vi "HEWH Agilent Create Label Array.vi"(8 "Error In":errorcluster, 9 "Agilent Calibrated Cluster Array":T1, 10 "Agilent Raw Cluster Array":T1, 11 "Label Array In":string[](array[string])) -> (0 "Error Out":errorcluster, 1 "Agilent Raw Cluster Array Out":T1, 2 "Agilent Calibrated Cluster Array In":T1, 3 "Label Array Out":string[](array[string]))   [LabVIEW 2016]
uses:
  Type Definitions/HEWH Agilent Cluster.ctl
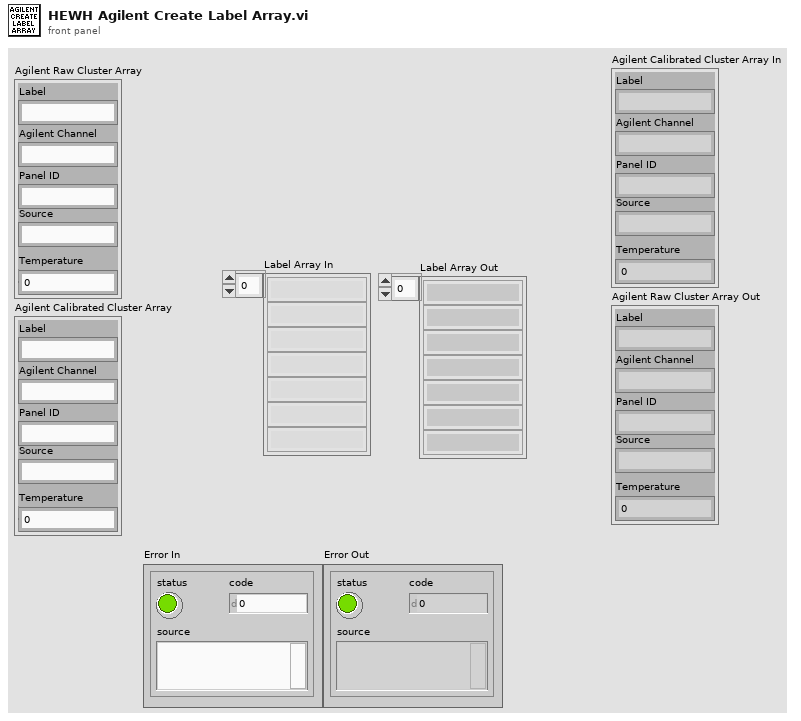
[diagram p1: front panel]
types:
  T1 = typedef "HEWH Agilent Cluster.ctl" = cluster{"Label":string, "Agilent Channel":string, "Panel ID":string, "Source":string, "Temperature":dbl}
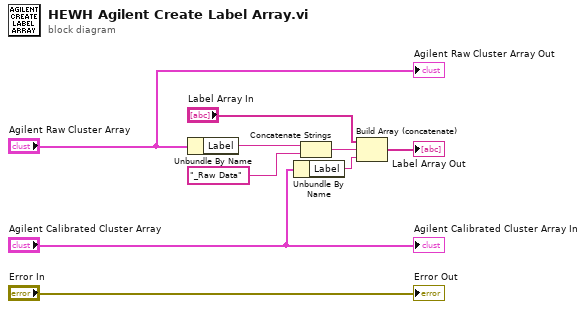
[diagram p0: block diagram]
diagram:
  n1 = Unbundle By Name("Agilent Raw Cluster Array") -> ("Label"=w6:string)
  n2 = Unbundle By Name("Agilent Calibrated Cluster Array") -> ("Label"=w3:string)
  n3 = Concatenate Strings(w6, "_Raw Data" ("string")) -> (w8:string)
  n4 = Build Array (concatenate)("Label Array In", w8, w3) -> (→"Label Array Out":string[])
  "Agilent Calibrated Cluster Array In" <- "Agilent Calibrated Cluster Array"
  "Agilent Raw Cluster Array Out" <- "Agilent Raw Cluster Array"
  "Error Out" <- "Error In"
